vi "Calculate conductance ITX.vi"(3 "single ended?":bool=TRUE, 4 "progress bar?":bool, 5 "length":i32=1, 7 "offset":i32, 9 "index":T2={"N1"=11, "N2"=19, "N3"=4, "N4"=5, "V1"=6, "V2"=4, "V3"=10, "V4"=13, "CURRENT"=7, "Vsg"=3}, 10 "File or Folder Path":path=path "P:/users1/kirkendall/data/SA02703M.20141112/7 - sweep Vsg, B") -> (0 "N Array":T1(array[cluster])=[{"N1"=0.0004, "N2"=0.0, "N3"=-6.47341032097701e-05, "N4"=-0.010645337299978234}], 1 "Comments":string="IGOR\nX// Date: 11/14/2014 5:01 PM\nX// SA02703M.20141112\nX// \nX// differential \nX// \nX// Vbg=-2.36V\nX// sweep Vsg: -100mV to 200mV, 1mV steps\nX// sweep B: sweep B 16T to -16T, 0.5T steps\nX// \nX// lockin\nX// 0: 3\nX// 1: 4, bad\nX// 2: 5\nX// 3: 7, curent \nX// 4: 9,\nX// 5: 2, current 5mV AC -190uV DC 400mHz\nX// appliedField= 16.000000\nX// appliedVsg= -0.100000\n\n\n\n\n\n\n\n\n\n\n\n\n\n\n\n\n\n\n\n\n\n\n\n\n\n\n\n\n\n\n\n\n\n\n\n\n\n\n\n\nX \nX Display/R 'time.SA02703M.20141112.0000'\nX AppendToGraph 'temp.SA02703M.20141112.0000'\nX AppendToGraph 'B.SA02703M.20141112.0000'\nX AppendToGraph 'Vsource.SA02703M.20141112.0000'\nX AppendToGraph 'Lockin0.SA02703M.20141112.0000'\nX AppendToGraph 'Lockin1.SA02703M.20141112.0000'\nX AppendToGraph 'Lockin2.SA02703M.20141112.0000'\nX AppendToGraph 'Lockin3.SA02703M.20141112.0000'\nX AppendToGraph 'Lockin4.SA02703M.20141112.0000'\nX AppendToGraph 'Lockin5.SA02703M.20141112.0000'\nX AppendToGraph 'B_rate.SA02703M.20141112.0000'\nX AppendToGraph 'DC0.SA02703M.20141112.0000'\nX AppendToGraph 'DC1.SA02703M.20141112.0000'\nX AppendToGraph 'DC2.SA02703M.20141112.0000'\nX AppendToGraph 'DC3.SA02703M.20141112.0000'\nX AppendToGraph 'DC4.SA02703M.20141112.0000'\nX AppendToGraph 'DC5.SA02703M.20141112.0000'\nX AppendToGraph 'DC6.SA02703M.20141112.0000'\nX AppendToGraph 'DC7.SA02703M.20141112.0000'\nX Label bottom \"x label\"\nX Label left \"y label\"\nX ModifyGraph rgb('time.SA02703M.20141112.0000')=(65280,0,0)\nX ModifyGraph rgb('temp.SA02703M.20141112.0000')=(65280,18432,0)\nX ModifyGraph rgb('B.SA02703M.20141112.0000')=(65280,36864,0)\nX ModifyGraph rgb('Vsource.SA02703M.20141112.0000')=(65280,55296,0)\nX ModifyGraph rgb('Lockin0.SA02703M.20141112.0000')=(57344,65280,0)\nX ModifyGraph rgb('Lockin1.SA02703M.20141112.0000')=(37376,65280,0)\nX ModifyGraph rgb('Lockin2.SA02703M.20141112.0000')=(18944,65280,0)\nX ModifyGraph rgb('Lockin3.SA02703M.20141112.0000')=(512,65280,0)\nX ModifyGraph rgb('Lockin4.SA02703M.20141112.0000')=(0,65280,17920)\nX ModifyGraph rgb('Lockin5.SA02703M.20141112.0000')=(0,65280,36352)\nX ModifyGraph rgb('B_rate.SA02703M.20141112.0000')=(0,65280,54784)\nX ModifyGraph rgb('DC0.SA02703M.20141112.0000')=(0,57856,65280)\nX ModifyGraph rgb('DC1.SA02703M.20141112.0000')=(0,39424,65280)\nX ModifyGraph rgb('DC2.SA02703M.20141112.0000')=(0,20992,65280)\nX ModifyGraph rgb('DC3.SA02703M.20141112.0000')=(0,2560,65280)\nX ModifyGraph rgb('DC4.SA02703M.20141112.0000')=(17408,0,65280)\nX ModifyGraph rgb('DC5.SA02703M.20141112.0000')=(35840,0,65280)\nX ModifyGraph rgb('DC6.SA02703M.20141112.0000')=(54272,0,65280)\nX ModifyGraph rgb('DC7.SA02703M.20141112.0000')=(65280,0,58368)\nX Legend/C/N=text0/J \"\\\\s('time.SA02703M.20141112.0000') time\\r\\\\s('temp.SA02703M.20141112.0000') temp\\r\\\\s('B.SA02703M.20141112.0000') B\\r\\\\s('Vsource.SA02703M.20141112.0000') Vsource\\r\\\\s('Lockin0.SA02703M.20141112.0000') Lockin0\\r\\\\s('Lockin1.SA02703M.20141112.0000') Lockin1\\r\\\\s('Lockin2.SA02703M.20141112.0000') Lockin2\\r\\\\s('Lockin3.SA02703M.20141112.0000') Lockin3\\r\\\\s('Lockin4.SA02703M.20141112.0000') Lockin4\\r\\\\s('Lockin5.SA02703M.20141112.0000') Lockin5\\r\\\\s('B_rate.SA02703M.20141112.0000') B_rate\\r\\\\s('DC0.SA02703M.20141112.0000') DC0\\r\\\\s('DC1.SA02703M.20141112.0000') DC1\\r\\\\s('DC2.SA02703M.20141112.0000') DC2\\r\\\\s('DC3.SA02703M.20141112.0000') DC3\\r\\\\s('DC4.SA02703M.20141112.0000') DC4\\r\\\\s('DC5.SA02703M.20141112.0000') DC5\\r\\\\s('DC6.SA02703M.20141112.0000') DC6\\r\\\\s('DC7.SA02703M.20141112.0000') DC7\"\nX ModifyGraph mirror(bottom)=1\nX ModifyGraph width=216\nX ModifyGraph height={Aspect,0.6}\nX ModifyGraph Log(bottom)=0\nX ModifyGraph Log(left)=0\nX \n", 2 "A vs D diff":cluster{dbl[], dbl[]}[](graph), 6 "angle phi":dbl[](array[numeric])=[179.65158969757934], 8 "angle theta":dbl[](array[numeric])=[-90.0], 11 "A vs D":cluster{dbl[], dbl[]}[](graph))   [LabVIEW 2016, in "Tranconductance SM.lvclass"]
uses:
  Tranconductance SM.lvclass
  <vilib>/Utility/miscctls.llb/LVOffsetAndMultiplierTypeDef.ctl
  <vilib>/addons/WireFlow/_WF_ProgressBar.llb/ProgressBar_WireFlow.lvclass
  <userlib>/LevyLab/XY Utilities/subVIs/Derivative (single).vi
  <userlib>/LevyLab/Graph Utilities/graph_utilities.lvclass
  <vilib>/Analysis/NI_AALPro.lvlib
  <userlib>/LevyLab/LV to ITX/Data/Data.lvclass
  <userlib>/LevyLab/XY Utilities/xy_utilities.lvlib
panel:
  out "WF-ProgressBar out":refnum<class "ProgressBar_WireFlow.lvclass">
  in  "Enum":enum16{"Conductance", "Resistance", "Current"}(ring)
  in  "alpha":dbl=0.00528086 format="%#_13g"
  in  "alpha?":bool
  in  "Numeric":dbl=50.0
  in  "Type":enum16{"dy/dx vs x", "dx/dy vs y"}(ring)
  in  "e^2/h?":bool=TRUE
  in  "log scale?":bool
  in  "calculate Ey":bool=TRUE
  in  "background":enum16{"do nothing", "subtract", "divide"}(ring)
  in  "Background":cluster{dbl[], dbl[]}[](graph)
  in  "A offset":dbl format="%#_6p"
  out "E 2":dbl[][](graph)
  out "counter":i32
  out "Path":path=path "P:/users1/kirkendall/data/SA02703M.20141112/7 - sweep Vsg, B/SA02703M.20141112.0000.itx"
  out "Index, Wavenames":string[][](table)=[["0", "'time.SA02703M.20141112.0000'\n"], ["1", "'temp.SA02703M.20141112.0000'\n"], ["2", "'B.SA02703M.20141112.0000'\n"], ["3", "'Vsource.SA02703M.20141112.0000'\n"], ["4", "'Lockin0.SA02703M.20141112.0000'\n"], ["5", "'Lockin1.SA02703M.20141112.0000'\n"], ["6", "'Lockin2.SA02703M.20141112.0000'\n"], ["7", "'Lockin3.SA02703M.20141112.0000'\n"], ["8", "'Lockin4.SA02703M.20141112.0000'\n"], ["9", "'Lockin5.SA02703M.20141112.0000'\n"], ["10", "'B_rate.SA02703M.20141112.0000'\n"], ["11", "'DC0.SA02703M.20141112.0000'\n"], ["12", "'DC1.SA02703M.20141112.0000'\n"], ["13", "'DC2.SA02703M.20141112.0000'\n"], ["14", "'DC3.SA02703M.20141112.0000'\n"], ["15", "'DC4.SA02703M.20141112.0000'\n"], ["16", "'DC5.SA02703M.20141112.0000'\n"], ["17", "'DC6.SA02703M.20141112.0000'\n"], ["18", "'DC7.SA02703M.20141112.0000'\n"], ["", ""]]
  out "N":cluster{"N1":dbl, "N2":dbl, "N3":dbl, "N4":dbl}={"N1"=0.0004, "N2"=0.0, "N3"=-6.47341032097701e-05, "N4"=-0.010645337299978234} {"N4" format="%#_6p"; "N3" format="%#_6p"; "N2" format="%#_6p"; "N1" format="%#_20p"}
  in  "Ey":T3={"Offset"=0.0, "Multiplier"=1.0}
  in  "Ex":T3={"Offset"=0.0, "Multiplier"=1.0}
  in  "recolor traces?":bool
  out "C vs D":cluster{dbl[], dbl[]}[](graph)
  out "E":dbl[][](graph)
  in  "B x name":string="Vsg (V)"
  in  "A y name":string="Conductance (S)"
  in  "Ex name":string="Ex name"
  in  "Ez name":string="Ez name"
  in  "D x name":string="Vsg (V)"
  in  "C y name":string="Conductance (S)"
  in  "Ey name":string="Ey name"
  out "time":string[][](table)=[["11/14/2014", "5:01 PM"]]
  in  "B is time?":bool
  in  "D  is time?":bool
  in  "pattern":string="*.itx"
  # "CURRENT/(V1-V2)"
  # "CURRENT/(V3-V4)"
  # "x axis: Vsg\ny axis: single ended?\nT: subtract V1-V2 and V3-V4 and divide by current\nF: plot V1/current"
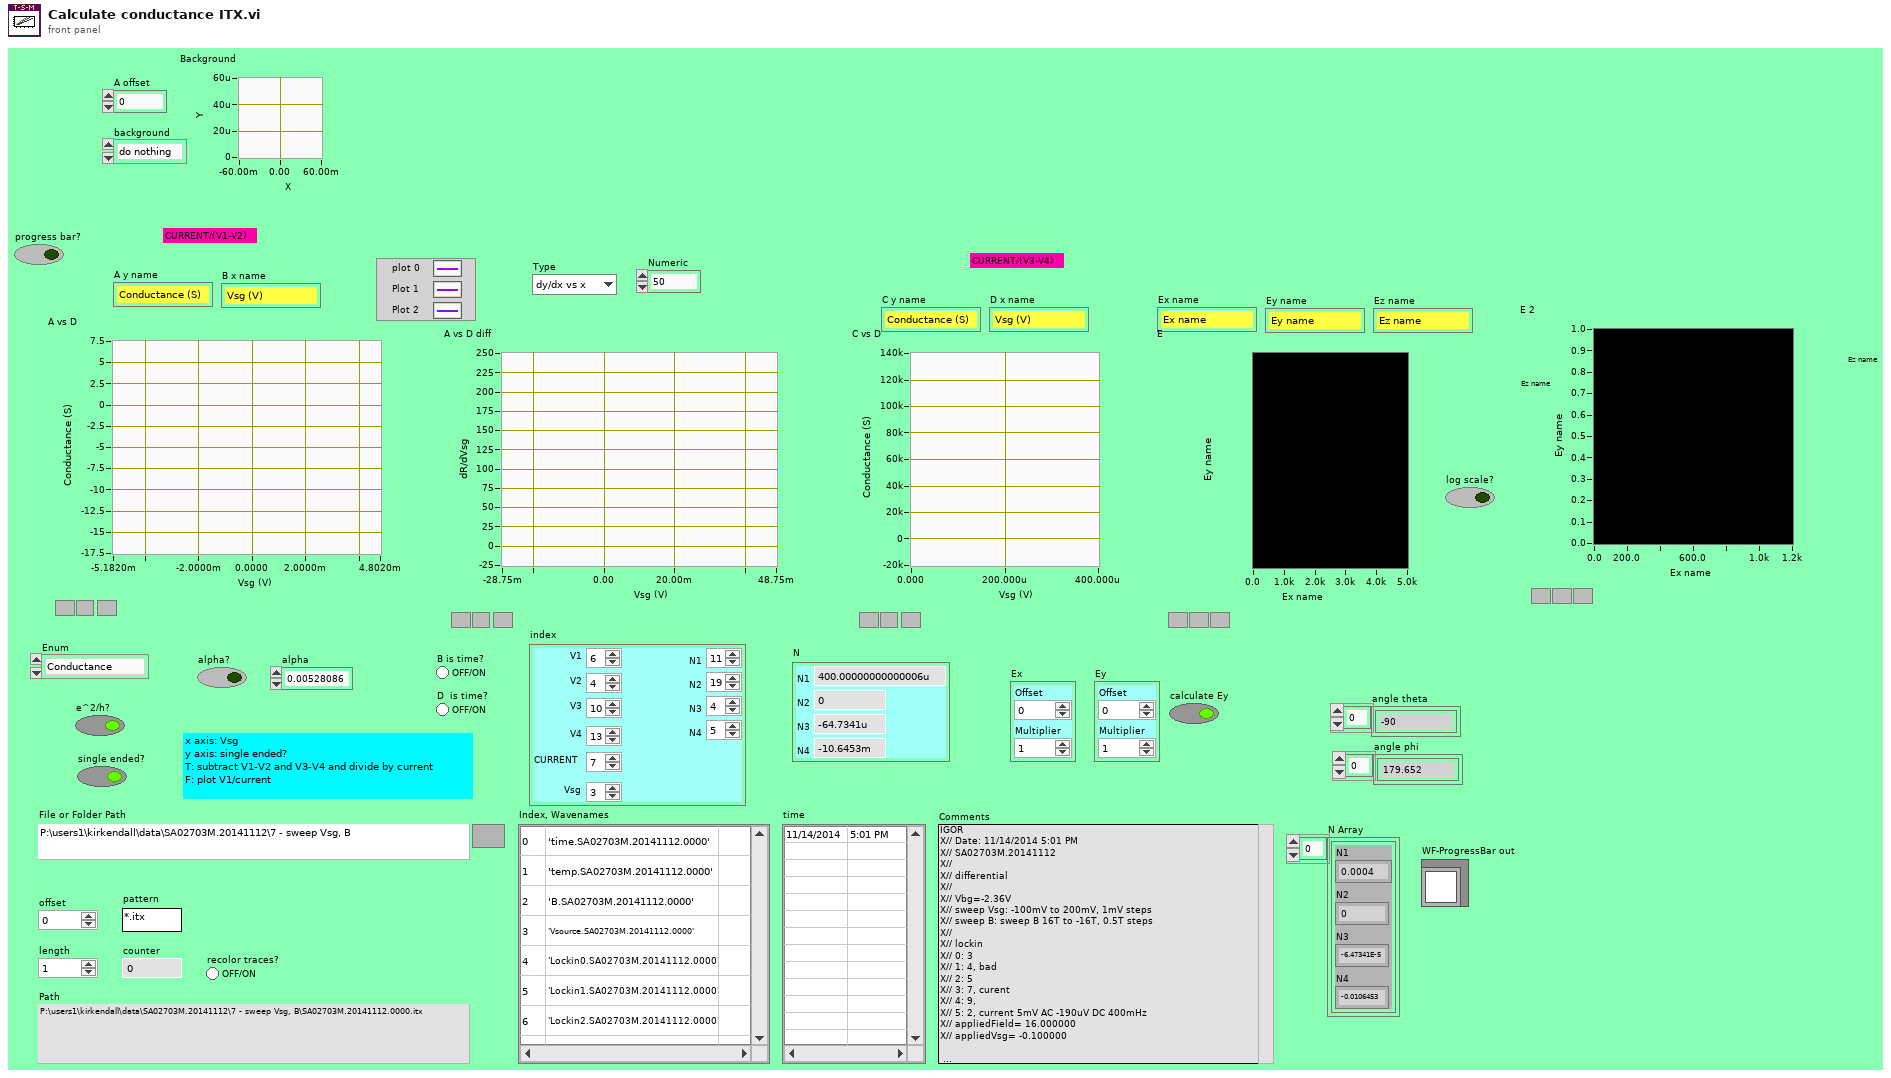
[diagram p1: front panel]
types:
  T1 = cluster{"N1":dbl, "N2":dbl, "N3":dbl, "N4":dbl}[]
  T2 = cluster{"N1":i32, "N2":i32, "N3":i32, "N4":i32, "V1":i32, "V2":i32, "V3":i32, "V4":i32, "CURRENT":i32, "Vsg":i32}
  T3 = typedef "LVOffsetAndMultiplierTypeDef.ctl" = cluster{"Offset":dbl, "Multiplier":dbl}
  T4 = typedef "Data.lvclass/Dictionary--cluster.ctl" = cluster{"key":string, "value":variant}
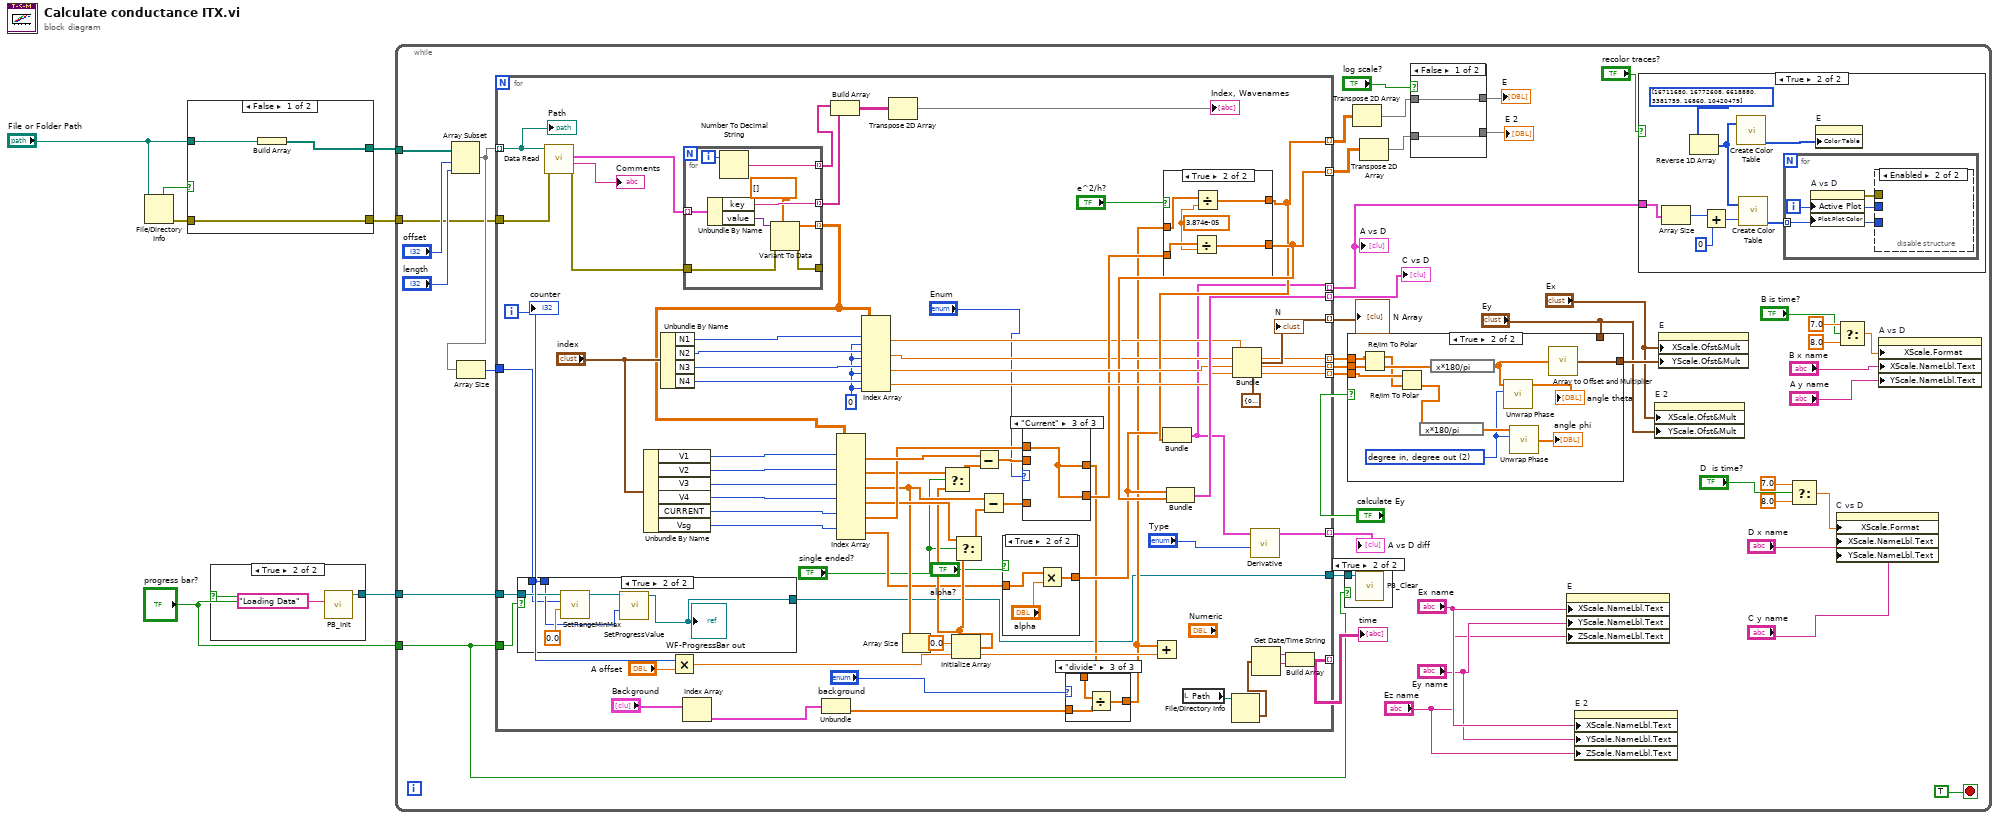
[diagram p0: block diagram]
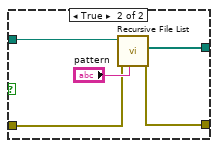
[diagram p2: hidden frame]
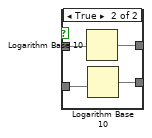
[diagram p5: hidden frame]
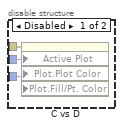
[diagram p8: hidden frame]
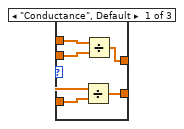
[diagram p12: hidden frame]
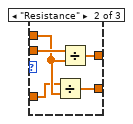
[diagram p13: hidden frame]
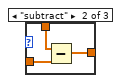
[diagram p15: hidden frame]
diagram:
  n1 = File/Directory Info(path="File or Folder Path") -> (directory=w2:bool, error out=w1:errorcluster)  [unwired: 1 in, 5 out]
  n2 = case shown="False" w2 {
    tunnel: [w10 w14] -> w6
    tunnel: "File or Folder Path" -> [w9 w13]
    tunnel: [w8 w11] -> w3
    tunnel: w1 -> [w8 w12]
    frame False {
      n3 = Build Array(w9) -> (w10:path[])
    }
    frame True {
      n4 = call <vilib>:"Recursive File List.vi"("pattern"="pattern", "error in (no error)"=w12, "Folder Path"=w13) -> ("error out"=w11:errorcluster, "All Files in Dir"=w14:path[])  [unwired: 4 in, 3 out]
    }
  }
  n5 = case shown="True" "progress bar?" {
    tunnel: [_ w17] -> w5
    frame False {
    }
    frame True {
      n6 = call <vilib>:"PB_Init.vi"("title (\"Progress\")"="Loading Data" ("title (\"Progress\")")) -> ("WF-ProgressBar out"=w17:refnum<class "ProgressBar_WireFlow.lvclass">)  [unwired: 9 in, 1 out]
    }
  }
  n7 = while {
    tunnel: w6 -> [w55]
    tunnel: w5 -> [w26]
    tunnel: "progress bar?" -> [w21]
    tunnel: w3 -> [w20]
    stop <- TRUE stop-if-true
    n8 = Array Subset(array=w55, index="offset", length="length") -> (w24:path[])
    n9 = Array Size(array=w24) -> (size(s)=w23:i32)
    n10 = for {
      tunnel: w24 -> [w167] mode=indexing
      tunnel: [w167] -> _ mode=indexing
      tunnel: [w155] -> w57 mode=indexing
      tunnel: [w99] -> w46 mode=indexing
      tunnel: [w143] -> w47 mode=indexing
      tunnel: [w130] -> w45 mode=indexing
      tunnel: [w131] -> w44 mode=indexing
      tunnel: [w119] -> w39 mode=indexing
      tunnel: [w135] -> w38 mode=indexing
      tunnel: [w134] -> w37 mode=indexing
      tunnel: [w129] -> w28 mode=indexing
      tunnel: [w98] -> w27 mode=indexing
      tunnel: w26 -> [w111]
      tunnel: w23 -> [w109]
      tunnel: [w108] -> w22
      tunnel: w21 -> [w107]
      tunnel: w20 -> [w104]
      i -> [w110]
      w153 = 0 ("disabled index (col)")
      n11 = case shown="True" w107 {
        tunnel: w111 -> [_ w182]
        tunnel: w110 -> [_ w179]
        tunnel: w109 -> [_ w178]
        tunnel: [_ w177] -> w108
        frame False {
        }
        frame True {
          n12 = call-dynamic "SetRangeMinMax.vi"("Min (0)"=0.0, "Max (1)"=w178, "WF-ProgressBar in"=w182) -> ("WF-ProgressBar out"=w180:refnum<class "ProgressBar_WireFlow.lvclass">)  [unwired: 7 in, 1 out]
          n13 = call-dynamic "SetProgressValue.vi"("Value"=w179, "WF-ProgressBar in"=w180) -> ("WF-ProgressBar out"=w177:refnum<class "ProgressBar_WireFlow.lvclass">)  [unwired: 7 in, 2 out]
          "WF-ProgressBar out" <- w177
        }
      }
      n14 = call <userlib>:"Data Read.vi"("error in (no error)"=w104, "path"=w167) -> ("error out"=w103:errorcluster, "Notes"=→"Comments":string, "Data (Dictionary)"=w106:T4[])  [unwired: 6 in, 1 out]
      n15 = Unbundle By Name("index") -> ("V1"=w152:i32, "V2"=w151:i32, "V3"=w150:i32, "V4"=w149:i32, "CURRENT"=w147:i32, "Vsg"=w142:i32)
      n16 = Unbundle By Name("index") -> ("N1"=w160:i32, "N2"=w161:i32, "N3"=w162:i32, "N4"=w163:i32)
      n17 = Multiply(x=w110, y="A offset") -> (x*y=w140:dbl)
      n18 = Index Array(array="Background") -> (element=w137:cluster{dbl[], dbl[]})  [unwired: 1 in]
      n19 = for {
        tunnel: [w175] -> w101 mode=indexing
        tunnel: w106 -> [w174] mode=indexing
        tunnel: [w173] -> w102 mode=indexing
        tunnel: [w171] -> w105 mode=indexing
        tunnel: w103 -> [w169]
        tunnel: [w168] -> _
        i -> [w176]
        n20 = Unbundle By Name(w174) -> ("key"=w173:string, "value"=w170:variant)
        n21 = Number To Decimal String(number=w176) -> (decimal integer string=w175:string)  [unwired: 1 in]
        n22 = Variant To Data(error in=w169, type=dbl[] [], Variant=w170) -> (data=w171:dbl[], error out=w168:errorcluster)
      }
      n23 = Unbundle(w137) -> (w138:dbl[])  [unwired: 1 out]
      n24 = Build Array(w101, w102) -> (w165:string[][])
      n25 = Index Array(array=w105, index (row) #1=w152, index (row) #2=w151, index (row) #3=w150, index (row) #4=w149, index (row) #5=w147, index (row) #6=w142) -> (element #1=w148:dbl[], element #2=w128:dbl[], element #3=w124:dbl[], element #4=w126:dbl[], element #5=w145:dbl[], element #6=w117:dbl[])  [unwired: 6 in]
      n26 = Index Array(array=w105, index (row) #1=w160, index (col) #1=w153, index (row) #2=w161, index (col) #2=w153, index (row) #3=w162, index (col) #3=w153, index (row) #4=w163, index (col) #4=w153) -> (element #1=w120:dbl, element #2=w119:dbl, element #3=w135:dbl, element #4=w134:dbl)
      n27 = Transpose 2D Array(2D array=w165) -> (transposed array=→"Index, Wavenames":string[][])
      n28 = Array Size(array=w124) -> (size(s)=w122:i32)
      n29 = Initialize Array(0.0 ("element"), w122) -> (w121:dbl[])
      n30 = Select(t=w128, s="single ended?", f=w121) -> (s? t:f=w127:dbl[])
      n31 = Select(t=w126, s="single ended?", f=w121) -> (s? t:f=w125:dbl[])
      n32 = Subtract(x=w148, y=w127) -> (x-y=w146:dbl[])
      n33 = Subtract(x=w124, y=w125) -> (x-y=w144:dbl[])
      n34 = case shown="True" "alpha?" {
        tunnel: w117 -> [w183 w186]
        tunnel: [w183 w185] -> w116
        frame False {
        }
        frame True {
          n35 = Multiply(x=w186, y="alpha") -> (x*y=w185:dbl[])
        }
      }
      n36 = case shown="\"Current\"" "Enum" {
        tunnel: w146 -> [w198 w203 _]
        tunnel: w145 -> [w197 w201 w204]
        tunnel: w144 -> [w196 w200 _]
        tunnel: [w195 w199 w204] -> w133
        tunnel: [w194 w202 w204] -> w114
        frame "Conductance", Default {
          n37 = Divide(x=w197, y=w196) -> (x/y=w195:dbl[])
          n38 = Divide(x=w197, y=w198) -> (x/y=w194:dbl[])
        }
        frame "Resistance" {
          n39 = Divide(x=w200, y=w201) -> (x/y=w199:dbl[])
          n40 = Divide(x=w203, y=w201) -> (x/y=w202:dbl[])
        }
        frame "Current" {
        }
      }
      n41 = case shown="\"divide\"" "background" {
        tunnel: w114 -> [w205 w208 w211]
        tunnel: [w205 w207 w209] -> w115
        tunnel: w138 -> [_ w206 w210]
        frame "do nothing", Default {
        }
        frame "subtract" {
          n42 = Subtract(x=w208, y=w206) -> (x-y=w207:dbl[])
        }
        frame "divide" {
          n43 = Divide(x=w211, y=w210) -> (x/y=w209:dbl[])
        }
      }
      n44 = Add(x=w115, y=w140) -> ()  [unwired: 1 out]
      n45 = case shown="True" "e^2/h?" {
        tunnel: w133 -> [w187 w191]
        tunnel: w115 -> [w188 w193]
        tunnel: [w188 w192] -> w130
        tunnel: [w187 w190] -> w131
        frame False {
        }
        frame True {
          w189 = 3.874e-05
          n46 = Divide(x=w191, y=w189) -> (x/y=w190:dbl[])
          n47 = Divide(x=w193, y=w189) -> (x/y=w192:dbl[])
        }
      }
      n48 = Bundle(w116, w130) -> (w99:cluster{dbl[], dbl[]})  [unwired: 1 in]
      n49 = Bundle(w116, w131) -> (w143:cluster{dbl[], dbl[]})  [unwired: 1 in]
      n50 = local read "Path"() -> (w159:path)
      n51 = File/Directory Info(path=w159) -> (last mod=w158:timestamp)  [unwired: 1 in, 6 out]
      n52 = Bundle(cluster=cluster{"N1":dbl, "N2":dbl, "N3":dbl, "N4":dbl} {"N1"=0.0, "N2"=0.0, "N3"=0.0, "N4"=0.0}, "N1"=w120, "N2"=w119, "N3"=w135, "N4"=w134) -> (w129:cluster{"N1":dbl, "N2":dbl, "N3":dbl, "N4":dbl})
      "N" <- w129
      n53 = call-poly <userlib>:"Derivative.vi"("Type"="Type", "XY-data"=w99) -> ("XY-data out"=w98:cluster{"X-array":dbl[], "Y-array":dbl[]})  [unwired: 7 in, 2 out]
      n54 = Get Date/Time String(seconds (now)=w158) -> (date string=w157:string, time string=w156:string)  [unwired: 2 in]
      n55 = Build Array(w157, w156) -> (w155:string[])
      "counter" <- w110
      "Path" <- w167
    }
    "A vs D" <- w46
    "C vs D" <- w47
    "time" <- w57
    "N Array" <- w28
    "A vs D diff" <- w27
    n56 = case shown="True" w21 {
      tunnel: w22 -> [_ w63]
      frame False {
      }
      frame True {
        n57 = call-dynamic "PB_Clear.vi"("WF-ProgressBar in"=w63) -> ()  [unwired: 9 in, 2 out]
      }
    }
    n58 = case shown="True" "calculate Ey" {
      tunnel: w39 -> [_ w82]
      tunnel: w38 -> [_ w81]
      tunnel: w37 -> [_ w76]
      tunnel: [w70 w74] -> w36
      tunnel: "Ey" -> [w70 _]
      frame False {
      }
      frame True {
        w72 = 2 items=["radian in, radian out", "radian in, degree out", "degree in, degree out", "degree in, radian out"] ("phase unit")
        n59 = Re/Im To Polar(2:w81, 3:w82) -> (0:w80:dbl[], 1:w75:dbl[])
        n60 = Re/Im To Polar(2:w75, 3:w76) -> (0:w71:dbl[])  [unwired: 1 out]
        n61 = expression code="x*180/pi"(w71) -> (w78:dbl[])
        n62 = expression code="x*180/pi"(w80) -> (w73:dbl[])
        n63 = call <vilib>:"Unwrap Phase.vi"("phase unit"=w72, "Phase"=w73) -> ("Unwrapped Phase"=→"angle theta":dbl[])  [unwired: 8 in, 1 out]
        n64 = call <vilib>:"Unwrap Phase.vi"("phase unit"=w72, "Phase"=w78) -> ("Unwrapped Phase"=→"angle phi":dbl[])  [unwired: 8 in, 1 out]
        n65 = call <userlib>:"Array to Offset and Multiplier.vi"("Array"=w73) -> ("Offset and Multiplier"=w74:T3)
      }
    }
    n66 = Transpose 2D Array(2D array=w45) -> (transposed array=w32:dbl[][])
    n67 = Transpose 2D Array(2D array=w44) -> (transposed array=w30:dbl[][])
    n68 = case shown="False" "log scale?" {
      tunnel: w32 -> [w65 w69]
      tunnel: [w65 w68] -> w31
      tunnel: w30 -> [w64 w67]
      tunnel: [w64 w66] -> w29
      frame False {
      }
      frame True {
        n69 = Logarithm Base 10(1:w69) -> (0:w68:dbl[][])
        n70 = Logarithm Base 10(1:w67) -> (0:w66:dbl[][])
      }
    }
    "E" <- w31
    "E 2" <- w29
    n71 = property on="E" class="IntGraph (strict)"("XScale.NameLbl.Text"="Ex name", "YScale.NameLbl.Text"="Ey name", "ZScale.NameLbl.Text"="Ez name") -> ()  [unwired: 2 in, 2 out]
    n72 = property on="E 2" class="IntGraph (strict)"("XScale.NameLbl.Text"="Ex name", "YScale.NameLbl.Text"="Ey name", "ZScale.NameLbl.Text"="Ez name") -> ()  [unwired: 2 in, 2 out]
    n73 = case shown="True" "recolor traces?" {
      tunnel: w46 -> [_ w83]
      frame False {
      }
      frame True {
        n74 = Array Size(array=w83) -> (size(s)=w86:i32)
        n75 = Reverse 1D Array(array=u32[] [16711680, 16772608, 6618880, 3381759, 16860, 10420479] ("color scale")) -> (reversed array=w85:u32[])
        n76 = Add(x=w86, y=0 ("x")) -> (x+y=w90:i32)
        n77 = call <userlib>:"Create Color Table.vi"("Colors []"=w85) -> ("Color Tbl"=w88:u32[])  [unwired: 1 in, 3 out]
        n78 = call <userlib>:"Create Color Table.vi"("Colors []"=w85, "Size (256)"=w90) -> ("Color Tbl"=w87:u32[])  [unwired: 3 out]
        n79 = for {
          tunnel: w87 -> [w91] mode=indexing
          i -> [w92]
          n80 = property on="A vs D" class="XYGraph (strict)"("Active Plot"=w92, "Plot.Plot Color"=w91) -> (error out=w93:errorcluster)  [unwired: 2 in, 1 out]
          n81 = disable-structure shown="Enabled" {
            disable-tunnel: w93 -> [w96 _]
            disable-tunnel: w92 -> [w95 _]
            disable-tunnel: w91 -> [w94 _]
            frame Disabled {
              n82 = property on="C vs D" class="XYGraph (strict)"(error in=w96, "Active Plot"=w95, "Plot.Plot Color"=w94, "Plot.Fill/Pt. Color"=w94) -> ()  [unwired: 1 in, 2 out]
            }
            frame Enabled {
            }
          }
        }
        n83 = property on="E" class="IntGraph (strict)"("Color Table"=w88) -> ()  [unwired: 2 in, 2 out]
      }
    }
    n84 = property on="E 2" class="IntGraph (strict)"("XScale.Ofst&Mult"="Ex", "YScale.Ofst&Mult"="Ey") -> ()  [unwired: 2 in, 2 out]
    n85 = property on="E" class="IntGraph (strict)"("XScale.Ofst&Mult"="Ex", "YScale.Ofst&Mult"=w36) -> ()  [unwired: 2 in, 2 out]
    n86 = Select(t=7.0, s="D  is time?", f=8.0) -> (s? t:f=w51:dbl)
    n87 = property on="C vs D" class="XYGraph (strict)"("XScale.Format"=w51, "XScale.NameLbl.Text"="D x name", "YScale.NameLbl.Text"="C y name") -> ()  [unwired: 2 in, 2 out]
    n88 = Select(t=7.0, s="B is time?", f=8.0) -> (s? t:f=w52:dbl)
    n89 = property on="A vs D" class="XYGraph (strict)"("XScale.Format"=w52, "XScale.NameLbl.Text"="B x name", "YScale.NameLbl.Text"="A y name") -> ()  [unwired: 2 in, 2 out]
  }
